vi "test.workspace_create_datasource_without_workspace.vi"   [LabVIEW 2020]
uses:
  Nominal Client/Nominal Client.lvclass/Nominal Client.ctl
  d8fc6ebf-c21d-4830-bd1f-6c9a88ac88e5.vi
  Nominal Client/private_data.set.vi
  <vilib>/Utility/error.llb/Error Cluster From Error Code.vi
  submodules/reqwest-labview/lv-src/reqwest/create.vi
  <vilib>/addons/_JKI Toolkits/Caraya/classes/Assert/Assert Error.vi
  Nominal Client/Nominal Client.lvclass
  nominal types/workspace/workspace.lvclass
  submodules/reqwest-labview/lv-src/reqwest/reqwest.lvclass
  <vilib>/addons/_JKI Toolkits/Caraya/classes/Assert/Assert.lvclass
  <vilib>/addons/_JKI Toolkits/Caraya/classes/Test/Test.lvclass
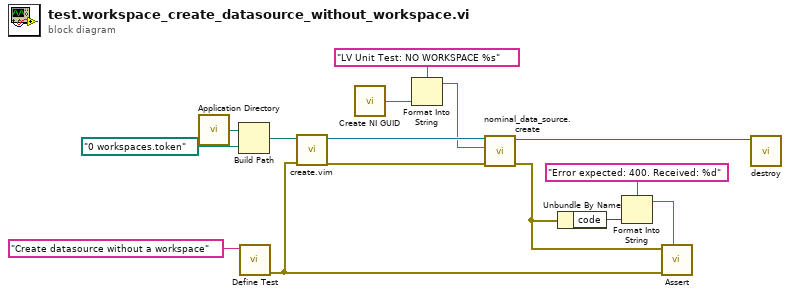
[diagram p0: block diagram]
diagram:
  n1 = call <vilib>:"Application Directory.vi"() -> ("Application Directory"=w14:path)
  n2 = Build Path(base path=w14, name or relative path=path "0 workspaces.token" ("Path")) -> (appended path=w15:path)
  n3 = call <vilib>:"Define Test.vi"("Label (VI Title)"="Create datasource without a workspace") -> ("error out"=w5:errorcluster)  [unwired: 9 in, 1 out]
  n4 = call "create.vim"("error in"=w5, "API Token (string or path)"=w15) -> ("error out"=w8:errorcluster, "Nominal Client"=w10:refnum<class "Nominal Client.lvclass">)  [unwired: 8 in]
  n5 = call <vilib>:"Create NI GUID.vi"() -> ("NI GUID"=w11:string)
  n6 = Format Into String(format string="LV Unit Test: NO WORKSPACE %s", w11) -> (resulting string=w9:string)  [unwired: 2 in, 1 out]
  n7 = call "nominal_data_source.create.vi"("error in"=w8, "Name"=w9, "Nominal Client in"=w10) -> ("error out"=w2:errorcluster, "Nominal Client out"=w6:refnum<class "Nominal Client.lvclass">)  [unwired: 5 in, 2 out]
  n8 = Unbundle By Name(w2) -> ("code"=w1:i32)
  n9 = Format Into String(format string="Error expected: 400. Received: %d" ("Label"), w1) -> (resulting string=w3:string)  [unwired: 2 in, 1 out]
  n10 = call-poly <vilib>:"Assert.vi"("Label"=w3, "error in (no error)"=w5, "Error?"=w2) -> ()  [unwired: 7 in, 2 out]
  n11 = call "destroy.vi"("Nominal Client"=w6) -> ()  [unwired: 10 in, 1 out]
